vi "RT LFO.vi"(6 "i":i32, 9 "freq":dbl=1.0 format="%0.2f") -> (1 "LFO Out":fxp<+/-,8,8>)   [LabVIEW 2015]
uses:
  <vilib>/ptbypt/NI_PtbyPt.lvlib
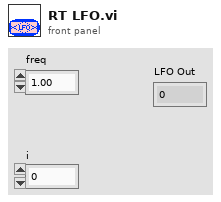
[diagram p1: front panel]
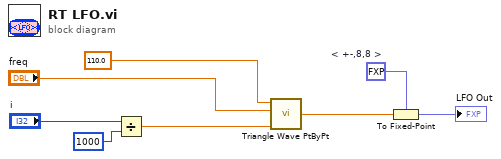
[diagram p0: block diagram]
diagram:
  w4 = fxp<+/-,8,8> 0.0  # < +-,8,8 >
  n1 = Divide(x="i", y=1000) -> (x/y=w7:dbl)
  n2 = call <vilib>:"Triangle Wave PtByPt.vi"("time"=w7, "frequency"="freq", "amplitude"=110.0 ("amp")) -> ("triangle wave"=w5:dbl)  [unwired: 1 in]
  n3 = To Fixed-Point(fixed-point type=w4, number=w5) -> (fixed-point=→"LFO Out":fxp<+/-,8,8>)
